vi "Fill Sylgard Dialog.vi"(8 "error in":errorcluster, 11 "Potting Procedure in":refnum<class "Potting Procedure.lvclass">) -> (0 "error out":errorcluster, 2 "Canceled":bool, 3 "Potting Procedure out":refnum<class "Potting Procedure.lvclass">)   [LabVIEW 2011]
uses:
  Procedure Classes/Potting Procedure/Potting Procedure.lvclass
  Shared Components/Gantry Class/Gantry Class.lvclass
  Shared Components/WorkTable Class/WorkTable Class.lvclass
panel:
  in  "OK Button":bool
  in  "Cancel Button":bool
  # "Now Mix some sylgard dummy!\nHere are instructions!\n    Step 1: Mix Sylgard\n    Step 2: ???\n    Step 3: Profit!\n\nClick \"OK\" when you are finished."
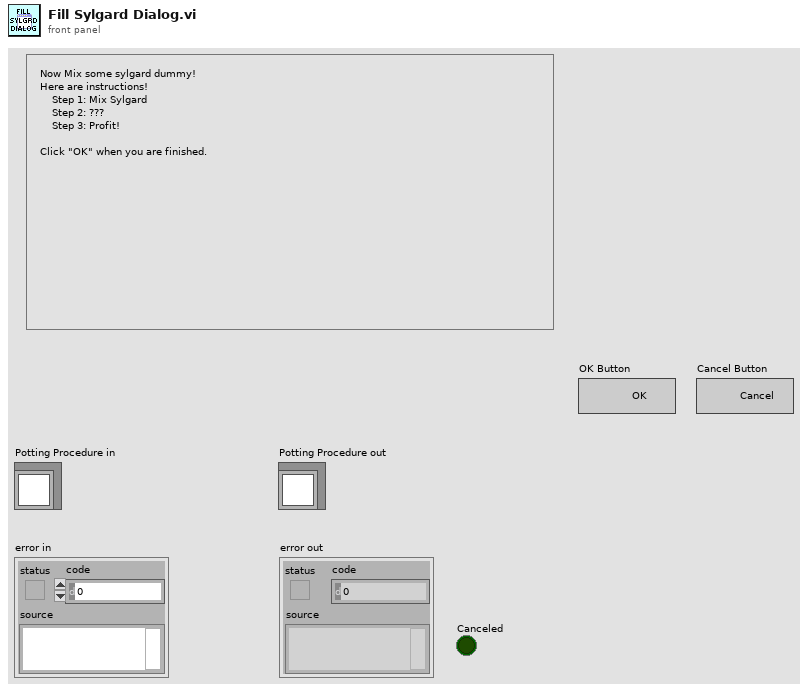
[diagram p1: front panel]
types:
  T1 = enum8{"Enabled", "Disabled", "Disabled and Grayed Out"}
  T2 = typedef "Worktable_Syringe.ctl" = cluster{"Syringe Holder":enum16{"Empty", "Populated", "Calibrated"}, "Mixing Time":timestamp, "Tip Offset":refnum<class "Vec3d Class.lvclass">}
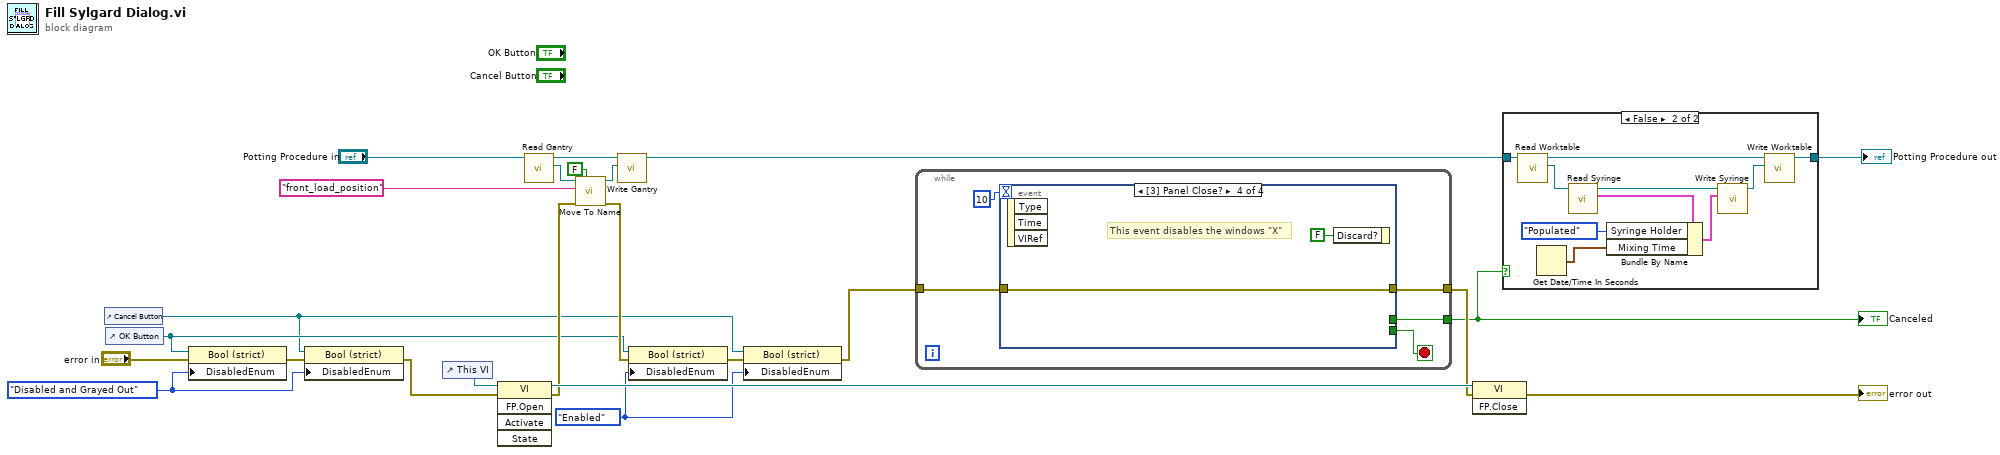
[diagram p0: block diagram]
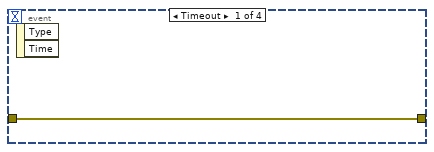
[diagram p3: hidden frame]
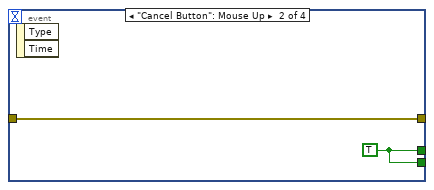
[diagram p4: hidden frame]
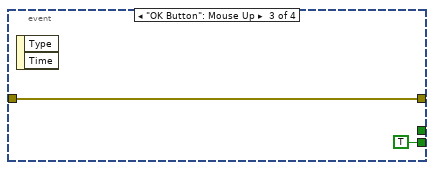
[diagram p5: hidden frame]
diagram:
  w1 = T1."Enabled" ("Disabled")
  w2 = T1."Disabled and Grayed Out" ("Disabled")
  n1 = control-ref of="Cancel Button"() -> (w3:refnum<vi>)
  n2 = control-ref of="OK Button"() -> (w4:refnum<vi>)
  n3 = property class="Bool (strict)"(reference=w4, error in="error in", "DisabledEnum"=w2) -> (error out=w9:errorcluster)  [unwired: 1 out]
  n4 = property class="Bool (strict)"(reference=w3, error in=w9, "DisabledEnum"=w2) -> (error out=w8:errorcluster)  [unwired: 1 out]
  n5 = control-ref of="This VI"() -> (w24:refnum<vi>)
  n6 = invoke class="VI" method="FP.Open"(reference=w24, error in=w8) -> (reference out=w23:refnum<vi>, error out=w16:errorcluster)  [unwired: 3 in, 3 out]
  n7 = call-dynamic "Read Gantry.vi"("Potting Procedure in"="Potting Procedure in") -> ("Gantry"=w19:refnum<class "Gantry Class.lvclass">, "Potting Procedure out"=w14:refnum<class "Potting Procedure.lvclass">)  [unwired: 8 in, 1 out]
  n8 = call-dynamic "Move To Name.vi"("Move if Same"=FALSE, "error in"=w16, "Destination Name"="front_load_position", "Gantry in"=w19) -> ("error out"=w6:errorcluster, "Gantry out"=w15:refnum<class "Gantry Class.lvclass">)  [unwired: 6 in]
  n9 = call-dynamic "Write Gantry.vi"("Gantry"=w15, "Potting Procedure in"=w14) -> ("Potting Procedure out"=w13:refnum<class "Potting Procedure.lvclass">)  [unwired: 8 in, 1 out]
  n10 = property class="Bool (strict)"(reference=w4, error in=w6, "DisabledEnum"=w1) -> (error out=w7:errorcluster)  [unwired: 1 out]
  n11 = property class="Bool (strict)"(reference=w3, error in=w7, "DisabledEnum"=w1) -> (error out=w5:errorcluster)  [unwired: 1 out]
  n12 = while {
    tunnel: [w25] -> w12
    tunnel: w5 -> [w26]
    tunnel: [w27] -> w21
    stop <- w28 stop-if-true
    n13 = event shown="[3] Panel Close?" {
      selector: _ -> [_ _ _ _]
      dyn-events: _ -> [_ _ _ _]
      timeout: 10 -> [_ _ _ _]
      tunnel: [_ w31 TRUE _] -> w28
      tunnel: [w30 w32 w34 w35] -> w27
      tunnel: w26 -> [w30 w32 w34 w35]
      tunnel: [_ w31 _ _] -> w25
      event Timeout {
        n14 = event-data() -> ()  [unwired: 1 in, 2 out]
      }
      event "Cancel Button": Mouse Up {
        w31 = TRUE
        n15 = event-data() -> ()  [unwired: 1 in, 2 out]
      }
      event "OK Button": Mouse Up {
        n16 = event-data() -> ()  [unwired: 1 in, 2 out]
      }
      event Panel Close? {
        # "This event disables the windows \"X\""
        n17 = event-data() -> ()  [unwired: 1 in, 3 out]
        n18 = event-data("Discard?"=FALSE) -> ()  [unwired: 1 in, 1 out]
      }
    }
  }
  "Canceled" <- w12
  n19 = invoke class="VI" method="FP.Close"(reference=w23, error in=w21) -> (error out=→"error out":errorcluster)  [unwired: 1 in, 2 out]
  n20 = case shown="False" w12 {
    tunnel: w13 -> [w37 w47]
    tunnel: [w37 w38] -> w11
    frame True {
    }
    frame False {
      n21 = call-dynamic "Read Worktable.vi"("Potting Procedure in"=w47) -> ("WorkTable out"=w46:refnum<class "WorkTable Class.lvclass">, "Potting Procedure out"=w39:refnum<class "Potting Procedure.lvclass">)  [unwired: 8 in, 1 out]
      n22 = Get Date/Time In Seconds() -> (seconds since 1Jan1904=w43:timestamp)
      n23 = call "Read Syringe.vi"("WorkTable in"=w46) -> ("Syringe"=w45:T2, "WorkTable out"=w42:refnum<class "WorkTable Class.lvclass">)  [unwired: 8 in, 1 out]
      n24 = Bundle By Name(cluster=w45, "Syringe Holder"=enum16{"Empty", "Populated", "Calibrated"}."Populated", "Mixing Time"=w43) -> (w41:T2)
      n25 = call-dynamic "Write Syringe.vi"("Syringe"=w41, "WorkTable Class in"=w42) -> ("WorkTable Class out"=w40:refnum<class "WorkTable Class.lvclass">)  [unwired: 8 in, 1 out]
      n26 = call-dynamic "Write Worktable.vi"("WorkTable in"=w40, "Potting Procedure in"=w39) -> ("Potting Procedure out"=w38:refnum<class "Potting Procedure.lvclass">)  [unwired: 8 in, 1 out]
    }
  }
  "Potting Procedure out" <- w11
